vi "Hardware - Analog Acquisition.vi"(7 "Terminated?":refnum<vi>, 8 "error in":errorcluster, 9 "SampClk.Timebase.Src":tag="/Dev3/PXI_Trig2", 10 "task/channels in":refnum<k21>="State System Analog Input", 11 "Named Data Structures":T1) -> (0 "error out":errorcluster)   [LabVIEW 2010, in "Core SubVIs.lvlib"]
doc: "This VI Creates the DAQ Counter Task for the System timer, sets up the analog input for triggered acquisition with the counter value as the timebase, then starts the analog input once the counter is armed.\n\nData is output to a Queue and the Counter Task is read independently.\n\nAccess data found in this VI using the following VIs:\nFor Counter Values: SubVIs\\Hardware - Counter Time.vi\nFor Analog Values: SubVIs\\Hardware - Access Analog Data Queue.vi"
uses:
  Core SubVIs.lvlib
  Controls/TYPE - Named Data Structures.ctl
  Controls/TYPE - Analog Data.ctl
  <vilib>/Utility/error.llb/DialogType.ctl
  Controls/TYPE - Count Time Method.ctl
  <vilib>/DAQmx/read.llb/DAQmx Read (Analog 1D Wfm NChan NSamp).vi
  <vilib>/daqmx/miscellaneous.llb/DAQmx Fill In Error Info.vi
  Program Files/National Instruments/LabVIEW 2010/resource/objmgr/daqmx.rc
panel:
  in  "number of samples per channel":i32=20
  out "AvailSampPerChan":u32
  out "Numeric":i32
  out "data":waveform(dbl)[](array[waveform])
  out "SampClk.TimebaseDiv":u32
  in  "stop":bool
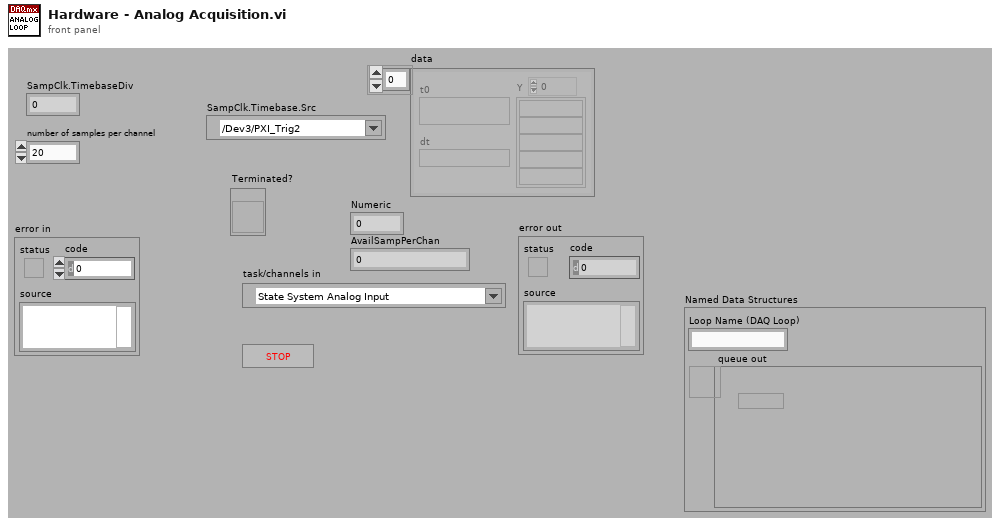
[diagram p1: front panel]
types:
  T1 = typedef "Core SubVIs.lvlib/TYPE - Named Data Structures.ctl" = cluster{"Loop Name (DAQ Loop)":string, "queue out":refnum<queue>}
  T2 = typedef "DialogType.ctl" = u16
  T3 = typedef "Core SubVIs.lvlib/TYPE - Count Time Method.ctl" = enum16{"Start Timer Task", "Read Timer", "Reset Timer", "Clear Timer Task"}
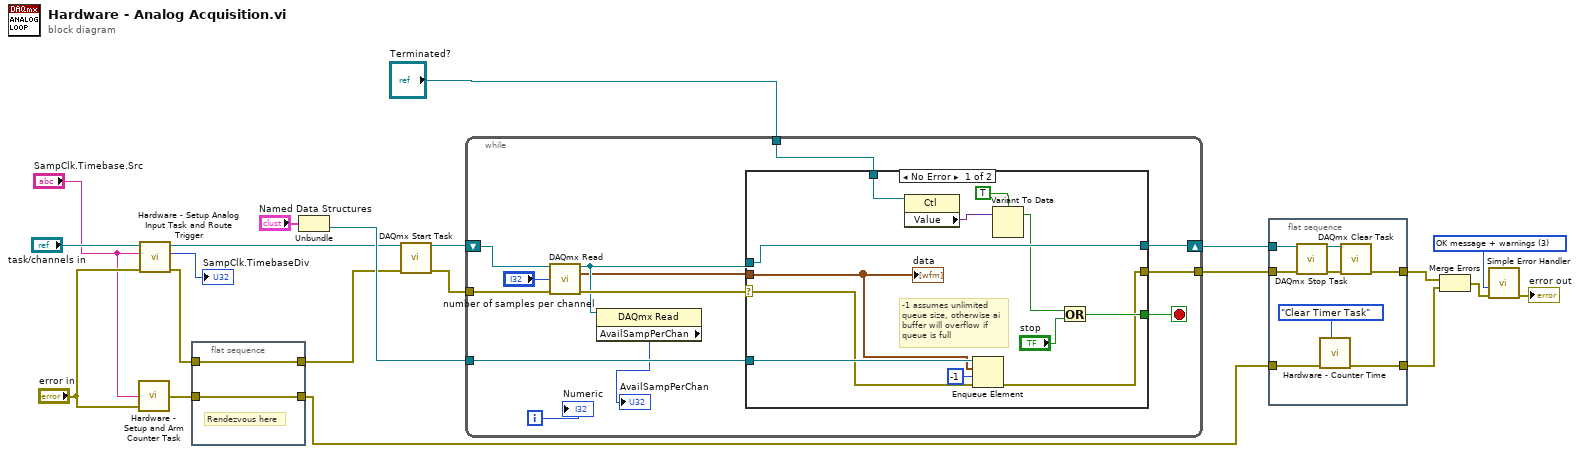
[diagram p0: block diagram]
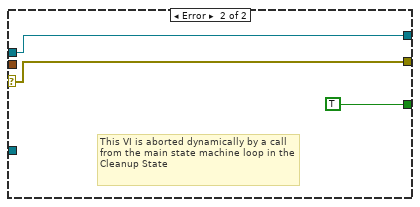
[diagram p2: hidden frame]
diagram:
  w19 = T2 3 items=["no dialog", "OK message", "continue or stop message", "OK message + warnings", "continue/stop + warnings"] ("type of dialog (OK msg:1)")
  n1 = call "Hardware - Setup and Arm Counter Task.vi"("error in"="error in", "CI.CountEdges.Term"="SampClk.Timebase.Src") -> ("error out"=w15:errorcluster)  [unwired: 1 in]
  n2 = call "Hardware - Setup Analog Input Task and Route Trigger.vi"("error in"="error in", "SampClk.Timebase.Src"="SampClk.Timebase.Src", "task/channels in"="task/channels in") -> ("error out"=w10:errorcluster, "SampClk.TimebaseDiv"=→"SampClk.TimebaseDiv":u32, "task out"=w5:refnum<k21>)  [unwired: 2 out]
  n3 = flat-sequence {
    tunnel: w10 -> [w23]
    tunnel: [w23] -> w14
    tunnel: w15 -> [w22]
    tunnel: [w22] -> w9
    frame #0 {
      # "Rendezvous here"
    }
  }
  n4 = Unbundle("Named Data Structures") -> ("queue out"=w16:refnum<queue>)  [unwired: 1 out]
  n5 = call <vilib>:"DAQmx Start Task.vi"("task/channels in"=w5, "error in"=w14) -> ("task out"=w20:refnum<k21>, "error out"=w21:errorcluster)  [unwired: 12 out]
  n6 = while {
    tunnel: w21 -> [w30]
    tunnel: w16 -> [w34]
    shift-right: [w27] -> w4
    shift-left: w20 -> [w31]
    tunnel: [w33] -> w3
    tunnel: "Terminated?" -> [w29]
    i -> [w35]
    stop <- w36 stop-if-true
    n7 = call-poly <vilib>:"DAQmx Read.vi"("task/channels in"=w31, "number of samples per channel"="number of samples per channel", "error in"=w30) -> ("task out"=w26:refnum<k21>, "data"=w24:waveform(dbl)[], "error out"=w28:errorcluster)  [unwired: 10 out]
    n8 = property class="DAQmx Read"(reference=w26) -> ("AvailSampPerChan"=→"AvailSampPerChan":u32)  [unwired: 1 in, 2 out]
    n9 = case shown="No Error" w28 {
      selector: w28 -> [w41 w49]
      tunnel: [w48 TRUE] -> w36
      tunnel: w26 -> [w42 w51]
      tunnel: [w42 w51] -> w27
      tunnel: [w44 w49] -> w33
      tunnel: w34 -> [w47 _]
      tunnel: w24 -> [w43 _]
      tunnel: w29 -> [w40 _]
      frame No Error {
        # "-1 assumes unlimited\nqueue size, otherwise ai\nbuffer will overflow if\nqueue is full"
        n10 = property class="Ctl"(reference=w40) -> ("Value"=w38:variant)  [unwired: 1 in, 2 out]
        n11 = Enqueue Element(queue=w47, element=w43, timeout in ms (-1)=-1, error in (no error)=w41) -> (error out=w44:errorcluster)  [unwired: 2 out]
        n12 = Variant To Data(Variant=w38, type=TRUE) -> (data=w37:bool)  [unwired: 1 in, 1 out]
        n13 = Or(x=w37, y="stop") -> (x .or. y?=w48:bool)
        "data" <- w43
      }
      frame Error {
        # "This VI is aborted dynamically by a call from the main state machine loop in the Cleanup State"
      }
    }
    "Numeric" <- w35
  }
  n14 = flat-sequence {
    tunnel: [w59] -> w8
    tunnel: w4 -> [w58]
    tunnel: w3 -> [w57]
    tunnel: w9 -> [w53]
    tunnel: [w52] -> w7
    frame #0 {
      n15 = call <vilib>:"DAQmx Stop Task.vi"("task/channels in"=w58, "error in"=w57) -> ("task out"=w56:refnum<k21>, "error out"=w55:errorcluster)  [unwired: 12 out]
      n16 = call "Hardware - Counter Time.vi"("Counter Time Function (Read Timer)"=TYPE_-_Count_Time_Method."Clear Timer Task", "error in (no error)"=w53) -> ("error out"=w52:errorcluster)  [unwired: 1 in, 8 out]
      n17 = call <vilib>:"DAQmx Clear Task.vi"("task in"=w56, "error in"=w55) -> ("error out"=w59:errorcluster)  [unwired: 13 out]
    }
  }
  n18 = Merge Errors(w8, w7) -> (w6:errorcluster)
  n19 = call <vilib>:"Simple Error Handler.vi"("type of dialog (OK msg:1)"=w19, "error in (no error)"=w6) -> ("error out"=→"error out":errorcluster)  [unwired: 7 out]
